vi "ack (SubVI).vi"() -> (2 "ACK":bool, 3 "SDA":bool)   [LabVIEW 2019]
uses:
  <vilib>/Platform/TimedLoop/XDataNode/timing_clust.ctl
  <vilib>/Platform/TimedLoop/XDataNode/nitl_modes.ctl
  <vilib>/Platform/TimedLoop/XDataNode/wakeup.ctl
  <vilib>/rvi/eio/common/nirviEmuTemplateMethod_errors.vi
  <vilib>/rvi/Emulation/niFpgaSctlEmulationGetInTimedLoop.vi
  <vilib>/rvi/Emulation/niFpgaEmulationReportErrorSimple.vi
  <vilib>/rvi/Emulation/niFpgaGetClockAttributes.vi
  <vilib>/rvi/Emulation/niFpgaCriticalErrorInLSC.vi
  <vilib>/eio/EIOMethodNode/EIOMethodNode.xnode
  <vilib>/eio/EIONode/EIONode.xnode
  <vilib>/platform/TimedLoop/XDataNode/XDataNode.xnode
  <vilib>/Platform/TimedLoop/XDataNode/XDNodeRunTimeDep.lvlib
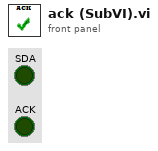
[diagram p1: front panel]
types:
  T1 = typedef "XDNodeRunTimeDep.lvlib/timing_clust.ctl" = cluster{"Expected End [f-1]":u64, "Actual End [f-1]":u64, "Finished Late? [f-1]":bool, "Expected End [i-1]":u64, "Actual End [i-1]":u64, "Finished Late? [i-1]":bool, "Expected Start [i]":u64, "Actual Start [i]":u64, "Expected Start [f]":u64, "Actual Start [f]":u64, "Source Name":string, "Structure Name":string, "Period":i64, "Deadline":i64, "Offset":i64, "Start":i64, "Priority":i32, "Timeout":i32, "Mode":T2, "Wakeup Reason":T3, "Error":errorcluster, "Source Type":string, "Secondary Source Type":string, "Global End Time":u64, "Global Start Time":u64, "Frame Duration":u64, "Iteration Duration":u64, "Assigned CPU":i32, "I/O Scan Engine Mode":u32}
  T2 = typedef "XDNodeRunTimeDep.lvlib/nitl_modes.ctl" = enum32{"No Change", "Process missed periods, maintain original phase", "Discard missed periods, maintain original phase", "Process missed periods, ignore original phase", "Discard missed periods, ignore original phase"}
  T3 = typedef "XDNodeRunTimeDep.lvlib/wakeup.ctl" = enum32{"Normal", "Aborted", "Asynchronous wakeup", "Timing source error", "Timed loop error", "Timeout"}
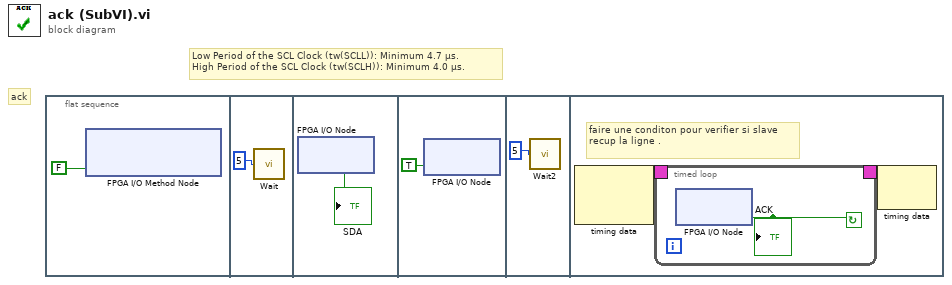
[diagram p0: block diagram]
diagram:
  # "Low Period of the SCL Clock (tw(SCLL)): Minimum 4.7 µs.\nHigh Period of the SCL Clock (tw(SCLH)): Minimum 4.0 µs."
  # "ack"
  n1 = flat-sequence {
    frame #0 {
      n2 = xnode "FPGA I/O Method Node"("Enable"=FALSE) -> ()  [unwired: 1 in, 1 out]
    }
    frame #1 {
      n3 = call "Wait"("Count(uSec)"=u32 5 ("Count(Ticks)")) -> ()  [unwired: 1 out]
    }
    frame #2 {
      n4 = xnode "FPGA I/O Node"() -> ("SDA"=→"SDA":bool)  [unwired: 1 in, 1 out]
    }
    frame #3 {
      n5 = xnode "FPGA I/O Node"("SCL"=TRUE) -> ()  [unwired: 1 in, 1 out]
    }
    frame #4 {
      n6 = call "Wait2"("Count(uSec)"=u32 5 ("Count(Ticks)")) -> ()  [unwired: 1 out]
    }
    frame #5 {
      # "faire une conditon pour verifier si slave recup la ligne ."
      n7 = node-c288() -> (w7:T1)  [unwired: 2 in]
      n8 = timed-loop {
        timing: w7 -> [_]
        timing-out: [_] -> w6
        stop <- w8 continue-if-true
        n9 = xnode "FPGA I/O Node"() -> ("SDA"=w8:bool)  [unwired: 1 in, 1 out]
        "ACK" <- w8
      }
      n10 = node-c288(w6) -> ()  [unwired: 1 out]
    }
  }
